vi "Initialize.vi"(8 "error in":errorcluster, 11 "Plugin in":refnum<class "Analog Tachometer Process.lvclass">) -> (0 "error out":errorcluster, 3 "Plugin out":refnum<class "Analog Tachometer Process.lvclass">)   [LabVIEW 2025, in "Analog Tachometer Process.lvlib" / "Analog Tachometer Process.lvclass"]
uses:
  Analog Tachometer Process.lvclass
  C:/Program Files/National Instruments/LabVIEW 2025/vi.lib/FlexLogger/SDK/PluginSDK.lvlibp/PEFClasses/SDK/Plugin/Plugin.lvclass
  <vilib>/FlexLogger/SDK/PluginSDK.lvlibp/PEFClasses/SDK/Processing Element/Timing Parameters.ctl
  <vilib>/FlexLogger/SDK/PluginSDK.lvlibp/PEFClasses/SDK/Processing Element/Timing Method.ctl
  <vilib>/FlexLogger/SDK/PluginSDK.lvlibp/PEFClasses/SDK/System Interface/Resampling Mode.ctl
  <vilib>/FlexLogger/SDK/PluginSDK.lvlibp/PEFClasses/SDK/Producer Channel/Producer Channel.lvclass
  C:/Program Files/National Instruments/LabVIEW 2025/vi.lib/FlexLogger/SDK/PluginSDK.lvlibp/PEFClasses/SDK/Channel/Channel.lvclass
  Helper VIs/Analog Tachometer Process Global.vi
  <vilib>/FlexLogger/SDK/PluginSDK.lvlibp/PEFClasses/SDK/Plugin/ParameterAccess/Write Command.vi
  <vilib>/FlexLogger/SDK/PluginSDK.lvlibp/PEFClasses/SDK/Plugin/ParameterAccess/Write Single Channel.vi
  <vilib>/FlexLogger/SDK/PluginSDK.lvlibp/PEFClasses/SDK/Plugin/ParameterAccess/Write I32.vi
  <vilib>/FlexLogger/SDK/PluginSDK.lvlibp/PEFClasses/SDK/Plugin/ParameterAccess/Write DBL.vi
  <vilib>/FlexLogger/SDK/PluginSDK.lvlibp/PEFClasses/SDK/Plugin/ParameterAccess/Write Enum.vi
  <vilib>/FlexLogger/SDK/PluginSDK.lvlibp/PEFClasses/SDK/Producer Channel/Create Producer Channel_v2.vi
  <vilib>/FlexLogger/SDK/PluginSDK.lvlibp/PEFClasses/SDK/Plugin/Plugin.lvclass
  C:/Program Files/National Instruments/LabVIEW 2025/vi.lib/FlexLogger/SDK/PluginSDK.lvlibp/PEFClasses/SDK/Processing Element/Processing Element.lvclass
  C:/dev/dsb/niflexlogger-plugins/PDK plugins/Analog Tachometer Process/source/Analog Tachometer Process/Analog Tachometer Process.lvclass
  <vilib>/FlexLogger/SDK/PluginSDK.lvlibp
  <vilib>/FlexLogger/SDK/PluginSDK.lvlibp/PEFClasses/SDK/Processing Element/Processing Element.lvclass
  <vilib>/FlexLogger/SDK/PluginSDK.lvlibp/PEFClasses/SDK/System Interface/System Interface.lvclass
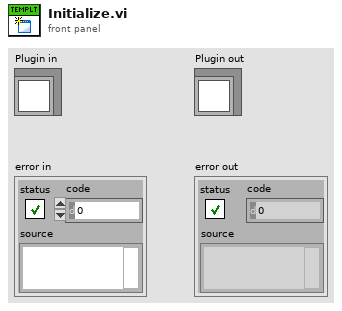
[diagram p1: front panel]
types:
  T1 = typedef "PluginSDK.lvlibp/System Interface.lvclass/Resampling Mode.ctl" = enum16{"No Resampling", "Custom Rate", "Maximum Rate", "Minimum Rate"}
  T2 = typedef "PluginSDK.lvlibp/Processing Element.lvclass/Timing Parameters.ctl" = cluster{"Timing Method":T3, "Timing Period (ms)":i32}
  T3 = typedef "PluginSDK.lvlibp/Processing Element.lvclass/Timing Method.ctl" = enum16{"Periodic", "Immediate", "On Data Ready", "Triggered"}
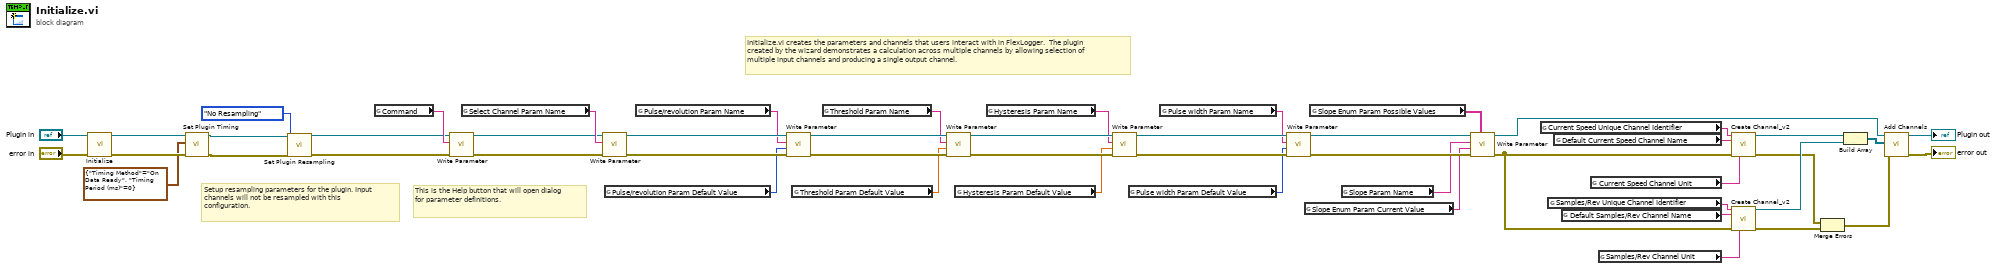
[diagram p0: block diagram]
diagram:
  # "This is the Help button that will open dialog for parameter definitions."
  # "Setup resampling parameters for the plugin. Input channels will not be resampled with this configuration."
  # "Initialize.vi creates the parameters and channels that users interact with in FlexLogger.  The plugin created by the wizard demonstrates a calculation across multiple channels by allowing selection of multiple input channels and producing a single output channel."
  n1 = call-parent "Initialize.vi"("error in (no error)"="error in", "Plugin in"="Plugin in") -> ("error out"=w48:errorcluster, "Plugin out"=w34:refnum<class "Analog Tachometer Process.lvclass">)  [unwired: 8 in]
  n2 = call <vilib>:"Set Plugin Timing.vi"("error in (no error)"=w48, "Timing Parameters"=T2 {"Timing Method"=enum."On Data Ready", "Timing Period (ms)"=0}, "Plugin in"=w34) -> ("error out"=w15:errorcluster, "Plugin out"=w16:refnum<class "Analog Tachometer Process.lvclass">)  [unwired: 7 in]
  n3 = call <vilib>:"Set Plugin Resampling.vi"("Plugin in"=w16, "Resampling Mode"=Resampling_Mode."No Resampling", "error in (no error)"=w15) -> ("Plugin out"=w2:refnum<class "Analog Tachometer Process.lvclass">, "error out"=w4:errorcluster)  [unwired: 11 in]
  n4 = global read "Analog Tachometer Process Global.vi" "Command"() -> (w3:string)
  n5 = call-poly <vilib>:"Write Parameter.vi"("error in (no error)"=w4, "Name"=w3, "Plugin in"=w2) -> ("error out"=w5:errorcluster, "Plugin out"=w6:refnum<class "Analog Tachometer Process.lvclass">)  [unwired: 7 in]
  n6 = global read "Analog Tachometer Process Global.vi" "Select Channel Param Name"() -> (w33:string)
  n7 = call-poly <vilib>:"Write Parameter.vi"("error in (no error)"=w5, "Name (Unique Channel Identifier)"=w33, "Plugin in"=w6) -> ("error out"=w43:errorcluster, "Plugin out"=w44:refnum<class "Analog Tachometer Process.lvclass">)  [unwired: 7 in]
  n8 = global read "Analog Tachometer Process Global.vi" "Pulse/revolution Param Default Value"() -> (w25:i32)
  n9 = global read "Analog Tachometer Process Global.vi" "Pulse/revolution Param Name"() -> (w32:string)
  n10 = call-poly <vilib>:"Write Parameter.vi"("error in (no error)"=w43, "Value"=w25, "Name"=w32, "Plugin in"=w44) -> ("error out"=w42:errorcluster, "Plugin out"=w41:refnum<class "Analog Tachometer Process.lvclass">)  [unwired: 6 in]
  n11 = global read "Analog Tachometer Process Global.vi" "Threshold Param Default Value"() -> (w24:dbl)
  n12 = global read "Analog Tachometer Process Global.vi" "Threshold Param Name"() -> (w31:string)
  n13 = call-poly <vilib>:"Write Parameter.vi"("error in (no error)"=w42, "Value"=w24, "Name"=w31, "Plugin in"=w41) -> ("error out"=w40:errorcluster, "Plugin out"=w39:refnum<class "Analog Tachometer Process.lvclass">)  [unwired: 6 in]
  n14 = global read "Analog Tachometer Process Global.vi" "Hysteresis Param Default Value"() -> (w22:dbl)
  n15 = global read "Analog Tachometer Process Global.vi" "Hysteresis Param Name"() -> (w30:string)
  n16 = call-poly <vilib>:"Write Parameter.vi"("error in (no error)"=w40, "Value"=w22, "Name"=w30, "Plugin in"=w39) -> ("error out"=w35:errorcluster, "Plugin out"=w36:refnum<class "Analog Tachometer Process.lvclass">)  [unwired: 6 in]
  n17 = global read "Analog Tachometer Process Global.vi" "Pulse width Param Default Value"() -> (w23:i32)
  n18 = global read "Analog Tachometer Process Global.vi" "Pulse width Param Name"() -> (w29:string)
  n19 = call-poly <vilib>:"Write Parameter.vi"("error in (no error)"=w35, "Value"=w23, "Name"=w29, "Plugin in"=w36) -> ("error out"=w38:errorcluster, "Plugin out"=w37:refnum<class "Analog Tachometer Process.lvclass">)  [unwired: 6 in]
  n20 = global read "Analog Tachometer Process Global.vi" "Slope Enum Param Current Value"() -> (w26:string)
  n21 = global read "Analog Tachometer Process Global.vi" "Slope Enum Param Possible Values"() -> (w28:string[])
  n22 = global read "Analog Tachometer Process Global.vi" "Slope Param Name"() -> (w27:string)
  n23 = call-poly <vilib>:"Write Parameter.vi"("Possible Values"=w28, "error in (no error)"=w38, "Current Value"=w26, "Name"=w27, "Plugin in"=w37) -> ("error out"=w7:errorcluster, "Plugin out"=w1:refnum<class "Analog Tachometer Process.lvclass">)  [unwired: 5 in]
  n24 = global read "Analog Tachometer Process Global.vi" "Current Speed Unique Channel Identifier"() -> (w21:string)
  n25 = global read "Analog Tachometer Process Global.vi" "Samples/Rev Unique Channel Identifier"() -> (w14:string)
  n26 = global read "Analog Tachometer Process Global.vi" "Default Current Speed Channel Name"() -> (w20:string)
  n27 = global read "Analog Tachometer Process Global.vi" "Default Samples/Rev Channel Name"() -> (w13:string)
  n28 = global read "Analog Tachometer Process Global.vi" "Current Speed Channel Unit"() -> (w19:string)
  n29 = global read "Analog Tachometer Process Global.vi" "Samples/Rev Channel Unit"() -> (w12:string)
  n30 = call-poly <vilib>:"Create Channel_v2.vi"("Unique Channel Identifier"=w21, "Default Channel Name"=w20, "error in (no error)"=w7, "Unit"=w19) -> ("Producer Channel"=w47:refnum<class "Producer Channel.lvclass">, "error out"=w8:errorcluster)  [unwired: 10 in]
  n31 = call-poly <vilib>:"Create Channel_v2.vi"("Unique Channel Identifier"=w14, "Default Channel Name"=w13, "error in (no error)"=w7, "Unit"=w12) -> ("Producer Channel"=w11:refnum<class "Producer Channel.lvclass">, "error out"=w9:errorcluster)  [unwired: 10 in]
  n32 = Merge Errors(w8, w9) -> (w10:errorcluster)
  n33 = Build Array(w47, w11) -> (w46:refnum<class "Producer Channel.lvclass">[])
  n34 = call <vilib>:"Add Channels.vi"("error in (no error)"=w10, "Channels"=w46, "Plugin in"=w1) -> ("error out"=→"error out":errorcluster, "Plugin out"=→"Plugin out":refnum<class "Analog Tachometer Process.lvclass">)  [unwired: 7 in]
